vi "Update List Options.vi"(8 "error in (no error)":errorcluster, 11 "List Data Type in":refnum<class "List Data Type.lvclass">) -> (0 "error out":errorcluster, 3 "List Data Type out":refnum<class "List Data Type.lvclass">)   [LabVIEW 2018, in "List Data Type.lvclass"]
uses:
  List Data Type.lvclass
  List Data Type.lvclass/List Data Type.ctl
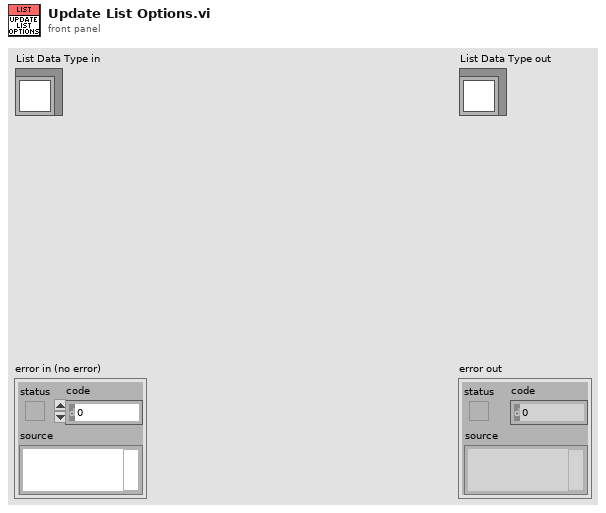
[diagram p1: front panel]
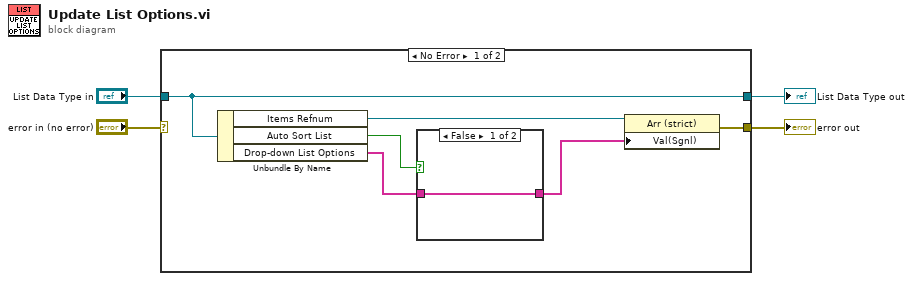
[diagram p0: block diagram]
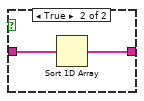
[diagram p2: hidden frame]
diagram:
  n1 = case shown="No Error" "error in (no error)" {
    selector: "error in (no error)" -> [_ w15]
    tunnel: [w5 w15] -> w3
    tunnel: [w10 w14] -> w1
    tunnel: "List Data Type in" -> [w10 w14]
    frame No Error {
      n2 = Unbundle By Name(w10) -> ("Items Refnum"=w9:refnum<vi>, "Auto Sort List"=w8:bool, "Drop-down List Options"=w7:string[])
      n3 = case shown="False" w8 {
        tunnel: w7 -> [w11 w13]
        tunnel: [w11 w12] -> w6
        frame False {
        }
        frame True {
          n4 = Sort 1D Array(array=w13) -> (sorted array=w12:string[])
        }
      }
      n5 = property class="Arr (strict)"(reference=w9, "Val(Sgnl)"=w6) -> (error out=w5:errorcluster)  [unwired: 1 in, 1 out]
    }
    frame Error {
    }
  }
  "error out" <- w3
  "List Data Type out" <- w1
